vi "FroLoop Get NCounter.vi"(1 "reference":refnum<vi>) -> (0 "ForLoopN":i32)   [LabVIEW 2014]
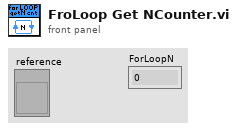
[diagram p1: front panel]
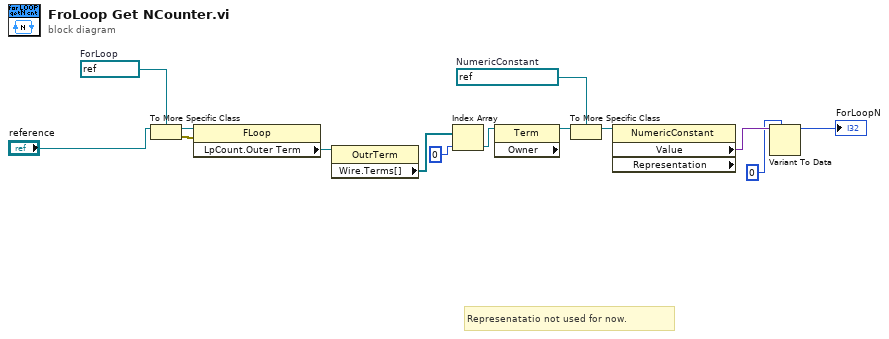
[diagram p0: block diagram]
diagram:
  w11 = refnum<vi> refnum  # NumericConstant
  w14 = refnum<vi> refnum  # ForLoop
  # "Represenatatio not used for now."
  n1 = To More Specific Class(target class=w14, reference="reference") -> (specific class reference=w13:refnum<vi>, error out=w12:errorcluster)  [unwired: 1 in]
  n2 = property class="FLoop"(reference=w13, error in=w12) -> ("LpCount.Outer Term"=w9:refnum<vi>)  [unwired: 2 out]
  n3 = property class="OutrTerm"(reference=w9) -> ("Wire.Terms[]"=w8:refnum<vi>[])  [unwired: 1 in, 2 out]
  n4 = Index Array(array=w8, index=0) -> (element=w6:refnum<vi>)
  n5 = property class="Term"(reference=w6) -> ("Owner"=w5:refnum<vi>)  [unwired: 1 in, 2 out]
  n6 = To More Specific Class(target class=w11, reference=w5) -> (specific class reference=w10:refnum<vi>)  [unwired: 1 in, 1 out]
  n7 = property class="NumericConstant" props=["Value", "Representation"](reference=w10) -> ("Value"=w4:variant)  [unwired: 1 in, 3 out]
  n8 = Variant To Data(type=0, Variant=w4) -> (data=→"ForLoopN":i32)  [unwired: 1 in, 1 out]
